vi "Merge Status.vi"(10 "New":T1, 11 "Current":T1) -> (3 "Merged":T1)   [LabVIEW 2020, in "Test Case Result.lvlib"]
uses:
  Test Case Result.lvlib
  Assertion Result/Public/TypeDefs/Status.ctl
  Assertion Result/Assertion Result.lvlib
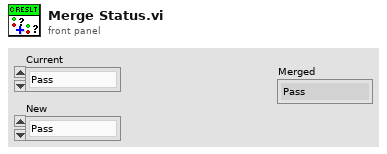
[diagram p1: front panel]
types:
  T1 = typedef "Assertion Result.lvlib/Status.ctl" = enum16{"Pass", "Fail", "Error", "Skipped", "Setup Error", "Broken", "Teardown Error"}
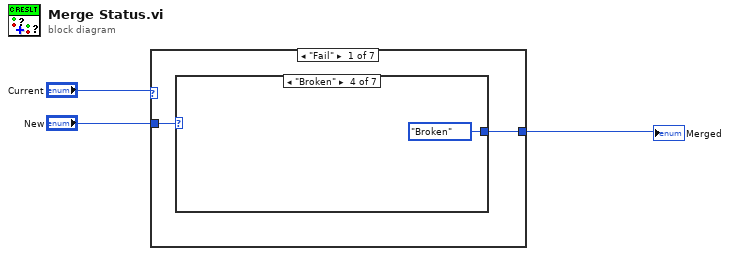
[diagram p0: block diagram]
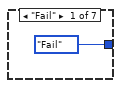
[diagram p2: hidden frame]
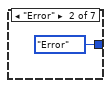
[diagram p3: hidden frame]
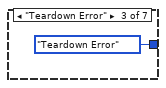
[diagram p4: hidden frame]
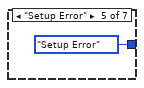
[diagram p5: hidden frame]
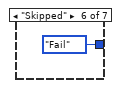
[diagram p6: hidden frame]
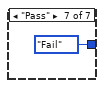
[diagram p7: hidden frame]
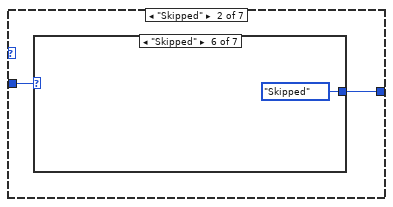
[diagram p8: hidden frame]
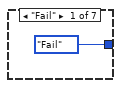
[diagram p9: hidden frame]
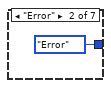
[diagram p10: hidden frame]
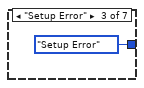
[diagram p11: hidden frame]
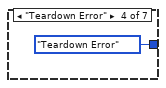
[diagram p12: hidden frame]
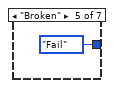
[diagram p13: hidden frame]
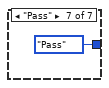
[diagram p14: hidden frame]
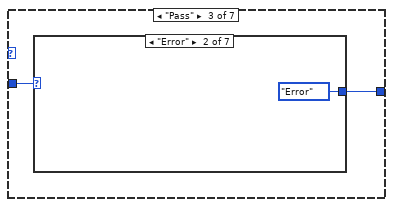
[diagram p15: hidden frame]
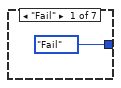
[diagram p16: hidden frame]
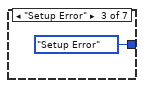
[diagram p17: hidden frame]
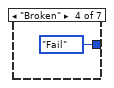
[diagram p18: hidden frame]
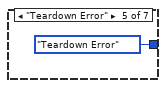
[diagram p19: hidden frame]
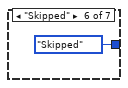
[diagram p20: hidden frame]
diagram:
  n1 = case shown="\"Fail\"" "Current" {
    tunnel: "New" -> [w5 w14 w23 _ _ w33 w37]
    tunnel: [w4 w13 w22 Status."Error" ("Merged Status") Status."Setup Error" ("Merged Status") w34 w37] -> w1
    frame "Fail" {
      n2 = case shown="\"Broken\"" w5 {
        tunnel: [Status."Fail" ("Merged Status") Status."Error" ("Merged Status") Status."Teardown Error" ("Merged Status") Status."Broken" ("Merged Status") Status."Setup Error" ("Merged Status") Status."Fail" ("Merged Status") Status."Fail" ("Merged Status")] -> w4
        frame "Fail" {
        }
        frame "Error" {
        }
        frame "Teardown Error" {
        }
        frame "Broken" {
        }
        frame "Setup Error" {
        }
        frame "Skipped" {
        }
        frame "Pass" {
        }
      }
    }
    frame "Skipped" {
      n3 = case shown="\"Skipped\"" w14 {
        tunnel: [Status."Fail" ("Merged Status") Status."Error" ("Merged Status") Status."Setup Error" ("Merged Status") Status."Teardown Error" ("Merged Status") Status."Fail" ("Merged Status") Status."Skipped" ("Merged Status") Status."Pass" ("Merged Status")] -> w13
        frame "Fail" {
        }
        frame "Error" {
        }
        frame "Setup Error" {
        }
        frame "Teardown Error" {
        }
        frame "Broken" {
        }
        frame "Skipped" {
        }
        frame "Pass" {
        }
      }
    }
    frame "Pass" {
      n4 = case shown="\"Error\"" w23 {
        tunnel: [Status."Fail" ("Merged Status") Status."Error" ("Merged Status") Status."Setup Error" ("Merged Status") Status."Fail" ("Merged Status") Status."Teardown Error" ("Merged Status") Status."Skipped" ("Merged Status") Status."Pass" ("Merged Status")] -> w22
        frame "Fail" {
        }
        frame "Error" {
        }
        frame "Setup Error" {
        }
        frame "Broken" {
        }
        frame "Teardown Error" {
        }
        frame "Skipped" {
        }
        frame "Pass" {
        }
      }
    }
    frame "Error" {
    }
    frame "Setup Error" {
    }
    frame "Teardown Error" {
      n5 = case shown="\"Error\", \"Setup Error\", \"Broken\"" w33 {
        selector: w33 -> [_ w36]
        tunnel: [Status."Teardown Error" ("Merged Status") w36] -> w34
        frame Default {
        }
        frame "Error", "Setup Error", "Broken" {
        }
      }
    }
    frame "Broken" {
    }
  }
  "Merged" <- w1
